vi "Ejercicio 1-5-6.vi"() -> ()   [LabVIEW 2013]
panel:
  in  "C o F":bool
  out "Temperatura convertida 2":dbl caption="[F]"
  in  "Temperatura a convertir":dbl caption="[C]"
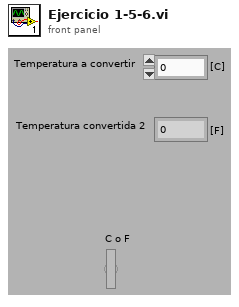
[diagram p1: front panel]
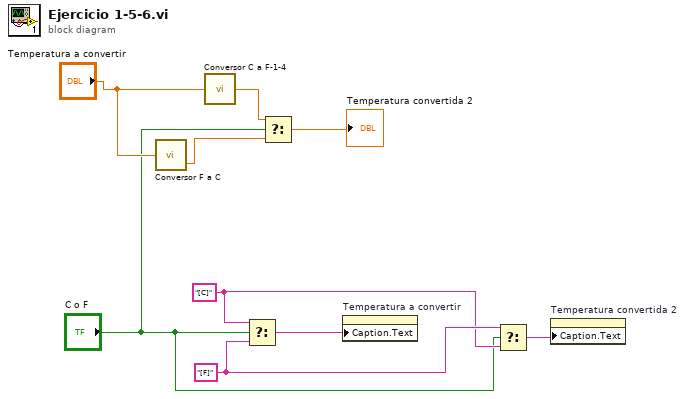
[diagram p0: block diagram]
diagram:
  w7 = "[F]"
  w6 = "[C]"
  n1 = call "Conversor F a C.vi"("Temperatura a convertir"="Temperatura a convertir") -> ("Temperatura convertida a F"=w3:dbl)  [unwired: 1 in]
  n2 = call "Conversor C a F-1-4.vi"("Temperatura a convertir"="Temperatura a convertir") -> ("Temp Convertida a C"=w4:dbl)
  n3 = Select(t=w6, s="C o F", f=w7) -> (s? t:f=w9:string)
  n4 = Select(t=w4, s="C o F", f=w3) -> (s? t:f=→"Temperatura convertida 2":dbl)
  n5 = property on="Temperatura a convertir" class="DigNum (strict)"("Caption.Text"=w9) -> ()  [unwired: 2 in, 2 out]
  n6 = Select(t=w7, s="C o F", f=w6) -> (s? t:f=w8:string)
  n7 = property on="Temperatura convertida 2" class="DigNum (strict)"("Caption.Text"=w8) -> ()  [unwired: 2 in, 2 out]
